vi "Self Queue Alias.vi"(11 "Queue in":refnum<class "Queue.lvclass">) -> (2 "Self Queue Alias":string)   [LabVIEW 2021, in "jettl.lvlib" / "Queue.lvclass"]
uses:
  Queue.lvclass
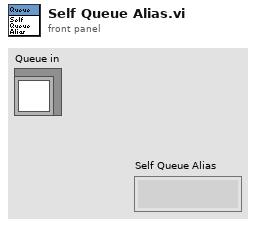
[diagram p1: front panel]
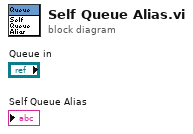
[diagram p0: block diagram]
diagram:
